vi "InitializeRoom.vi"(8 "error in (no error)":errorcluster, 10 "roomNumber":i32, 11 "Room in":refnum<class "Room.lvclass">) -> (0 "error out":errorcluster, 3 "Room out":refnum<class "Room.lvclass">)   [LabVIEW 2016, in "Room.lvclass"]
uses:
  Room.lvclass
  Room.lvclass/Room.ctl
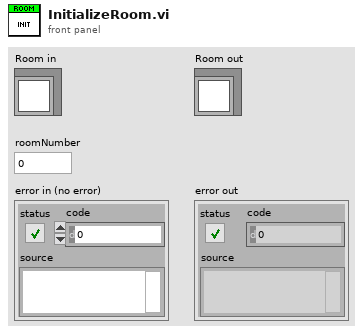
[diagram p1: front panel]
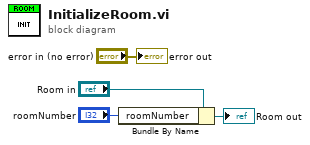
[diagram p0: block diagram]
diagram:
  n1 = Bundle By Name(cluster="Room in", "roomNumber"="roomNumber") -> (→"Room out":refnum<class "Room.lvclass">)
  "error out" <- "error in (no error)"
